vi "Read TDMS_Path.vi"(8 "error in (no error)":errorcluster, 11 "Report Viewer in":refnum<class "Report Viewer.lvclass">) -> (0 "error out":errorcluster, 2 "TDMS_Path":path, 3 "Report Viewer out":refnum<class "Report Viewer.lvclass">)   [LabVIEW 2019, in "Report Viewer.lvlib" / "Report Viewer.lvclass"]
uses:
  Library/Report Viewer.lvclass
  Library/Report Viewer.lvclass/Report Viewer.ctl
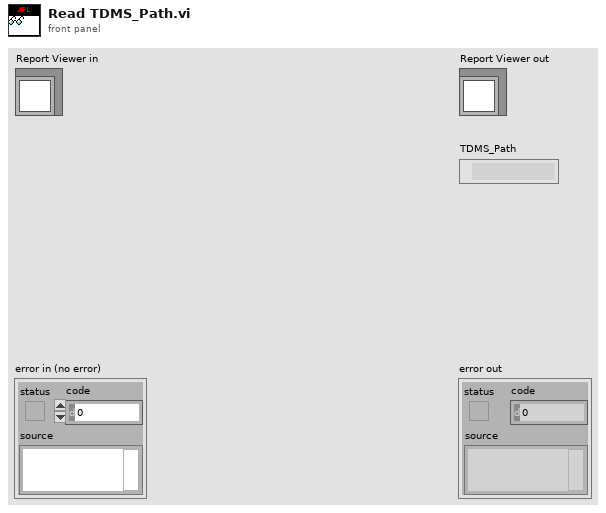
[diagram p1: front panel]
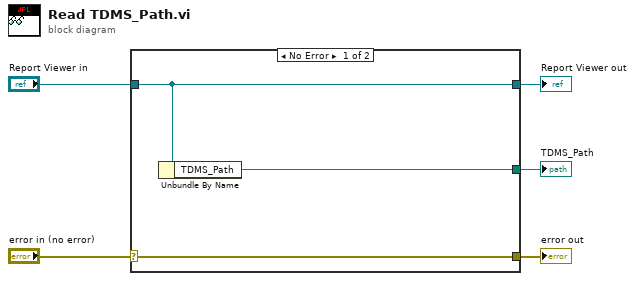
[diagram p0: block diagram]
diagram:
  n1 = case shown="No Error" "error in (no error)" {
    selector: "error in (no error)" -> [w8 w9]
    tunnel: [w8 w9] -> w4
    tunnel: [w7 w10] -> w2
    tunnel: "Report Viewer in" -> [w7 w10]
    tunnel: [w6 _] -> w1
    frame No Error {
      n2 = Unbundle By Name(w7) -> ("TDMS_Path"=w6:path)
    }
    frame Error {
    }
  }
  "error out" <- w4
  "Report Viewer out" <- w2
  "TDMS_Path" <- w1
